vi "Replace Formatting with Tags.vi"(7 "Set Value? (T)":bool, 8 "error in (no error)":errorcluster, 9 "Length":i32[](array[numeric]), 10 "Start":i32[](array[numeric]), 11 "Str Refnum":refnum<vi>) -> (0 "error out":errorcluster, 2 "New String":string, 3 "Str Refnum out":refnum<vi>)   [LabVIEW 2023, in "VI Properties Editor.lvlib"]
doc: "Replaces bold formatting with bold tags in the locations specified."
uses:
  VI Properties Editor.lvlib
  <vilib>/Utility/miscctls.llb/LVSelectionTypeDef.ctl
panel:
  out "Text.Selection End":u32
  out "Text.Selection Start":u32
  out "Text.Selection":T1
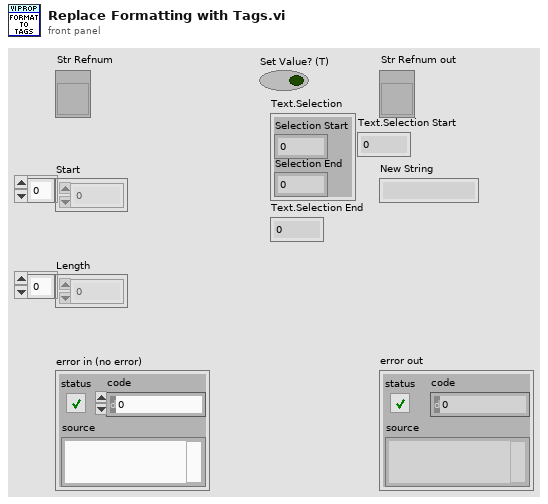
[diagram p1: front panel]
types:
  T1 = typedef "LVSelectionTypeDef.ctl" = cluster{"Selection Start":u32, "Selection End":u32}
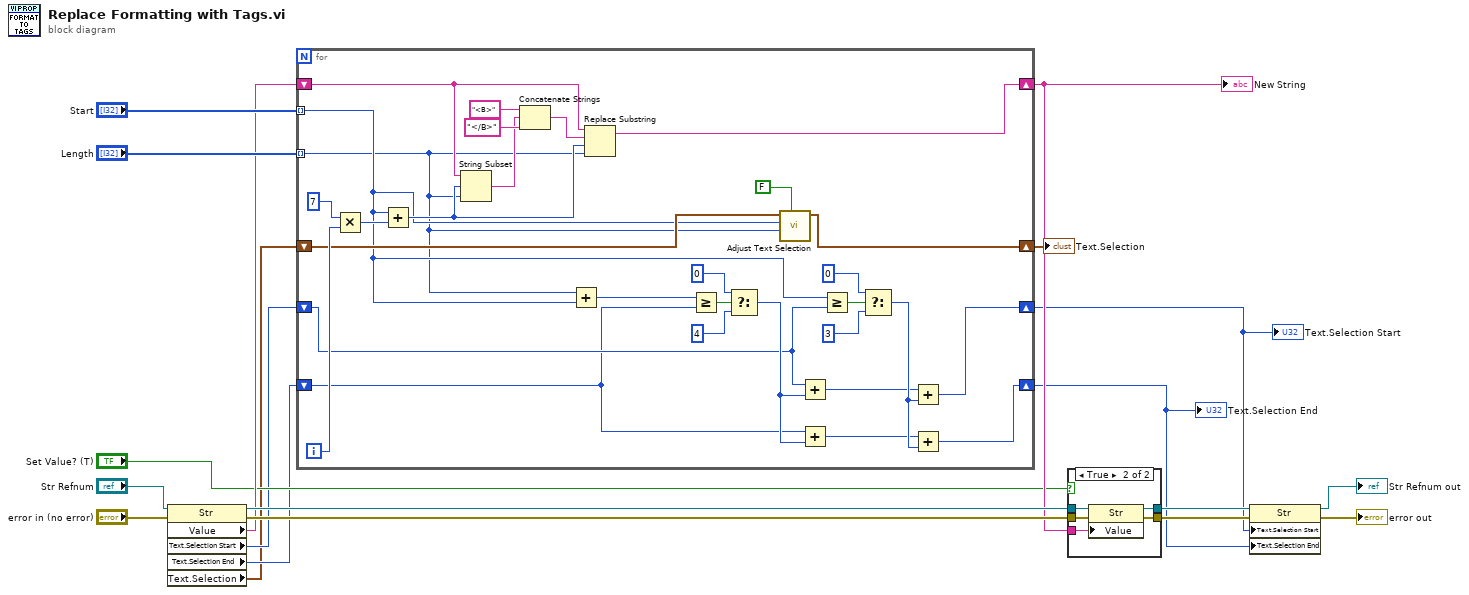
[diagram p0: block diagram]
diagram:
  n1 = property class="Str"(reference="Str Refnum", error in="error in (no error)") -> (reference out=w14:refnum<vi>, error out=w15:errorcluster, "Value"=w12:string, "Text.Selection Start"=w6:u32, "Text.Selection End"=w5:u32, "Text.Selection"=w2:T1)
  n2 = for {
    tunnel: "Length" -> [w22] mode=indexing
    tunnel: "Start" -> [w23] mode=indexing
    shift-right: [w46] -> w13
    shift-left: w12 -> [w41]
    shift-right: [w26] -> w3
    shift-left: w6 -> [w28]
    shift-right: [w25] -> w4
    shift-left: w5 -> [w27]
    shift-right: [w21] -> w1
    shift-left: w2 -> [w24]
    i -> [w44]
    n3 = Multiply(x=7, y=w44) -> (x*y=w42:i32)
    n4 = Add(x=w23, y=w42) -> (x+y=w40:i32)
    n5 = String Subset(string=w41, offset (0)=w40, length (rest)=w22) -> (substring=w47:string)
    n6 = Concatenate Strings("<B>" ("string"), w47, "</B>" ("string")) -> (w45:string)
    n7 = Add(x=w22, y=w23) -> (x+y=w29:i32)
    n8 = Replace Substring(2:w22, 3:w40, 4:w45, 5:w41) -> (1:w46:string)  [unwired: 1 out]
    n9 = Greater Or Equal?(x=w29, y=w27) -> (x >= y?=w34:bool)
    n10 = Select(t=u32 0 ("y"), s=w34, f=u32 4 ("y")) -> (s? t:f=w35:u32)
    n11 = call "Adjust Text Selection.vi"("Remove?"=FALSE, "Length"=w22, "Start"=w23, "Selection in"=w24) -> ("Selection out"=w21:T1)  [unwired: 7 in]
    n12 = Add(x=w28, y=w35) -> (x+y=w36:u32)
    n13 = Add(x=w27, y=w35) -> (x+y=w37:u32)
    n14 = Greater Or Equal?(x=w23, y=w28) -> (x >= y?=w38:bool)
    n15 = Select(t=u32 0 ("y"), s=w38, f=u32 3 ("y")) -> (s? t:f=w39:u32)
    n16 = Add(x=w36, y=w39) -> (x+y=w26:u32)
    n17 = Add(x=w37, y=w39) -> (x+y=w25:u32)
  }
  "New String" <- w13
  "Text.Selection" <- w1
  "Text.Selection Start" <- w3
  "Text.Selection End" <- w4
  n18 = case shown="True" "Set Value? (T)" {
    tunnel: w15 -> [w51 w56]
    tunnel: [w51 w55] -> w9
    tunnel: w14 -> [w50 w54]
    tunnel: [w50 w53] -> w10
    tunnel: w13 -> [_ w52]
    frame False {
    }
    frame True {
      n19 = property class="Str"(reference=w54, error in=w56, "Value"=w52) -> (reference out=w53:refnum<vi>, error out=w55:errorcluster)
    }
  }
  n20 = property class="Str"(reference=w10, error in=w9, "Text.Selection Start"=w3, "Text.Selection End"=w4) -> (reference out=→"Str Refnum out":refnum<vi>, error out=→"error out":errorcluster)
